vi "Port Number and Machine Name.vi"(0 "LV DEV in":refnum<class "LV DEV.lvclass">, 5 "PID":string, 11 "error in (no error)":errorcluster) -> (4 "LV DEV out":refnum<class "LV DEV.lvclass">, 6 "Machine Name":string, 8 "Port Number":u16, 15 "error out":errorcluster)   [LabVIEW 2016, in "LV DEV.lvclass"]
uses:
  LV DEV.lvclass
  <vilib>/regexp/Match Regular Expression.xnode
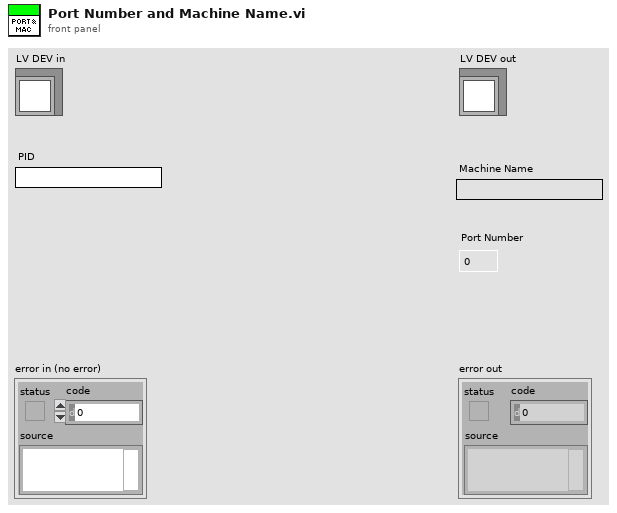
[diagram p1: front panel]
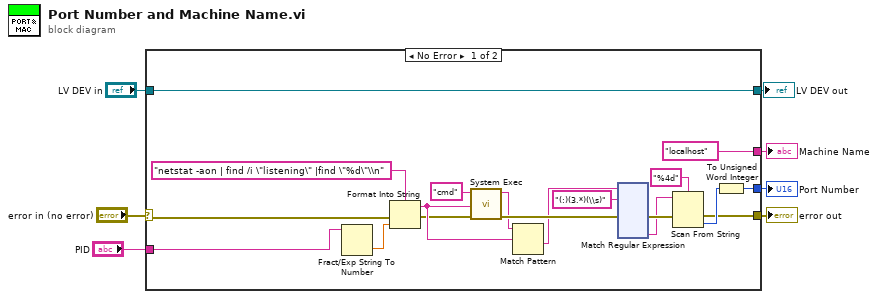
[diagram p0: block diagram]
diagram:
  n1 = case shown="No Error" "error in (no error)" {
    selector: "error in (no error)" -> [w12 w145]
    tunnel: [w11 w145] -> w6
    tunnel: "LV DEV in" -> [w26 w144]
    tunnel: [w26 w144] -> w4
    tunnel: "PID" -> [w10 _]
    tunnel: [w9 _] -> w2
    tunnel: ["localhost" _] -> w1
    frame No Error {
      n2 = Fract/Exp String To Number(string=w10) -> (number=w25:dbl)  [unwired: 3 in, 1 out]
      n3 = Format Into String(format string="netstat -aon | find /i \"listening\" |find \"%d\"\\n" ("standard input"), error in=w12, w25) -> (resulting string=w17:string, error out=w15:errorcluster)  [unwired: 1 in]
      n4 = call <vilib>:"System Exec.vi"("error in (no error)"=w15, "standard input"=w17, "command line"="cmd") -> ("error out"=w20:errorcluster, "standard output"=w16:string)  [unwired: 5 in, 2 out]
      n5 = Match Pattern(string=w16, regular expression=w17) -> (after substring=w18:string)  [unwired: 1 in, 3 out]
      n6 = xnode "Match Regular Expression"("input string"=w18, "regular expression"="(:)(3.*)(\\s)", "error in"=w20) -> ("error out"=w24:errorcluster, "submatch 2"=w21:string)  [unwired: 3 in, 5 out]
      n7 = Scan From String(format string="%4d", input string=w21, error in=w24) -> (error out=w11:errorcluster, output 1=w23:i32)  [unwired: 2 in, 2 out]
      n8 = To Unsigned Word Integer(number=w23) -> (unsigned 16bit integer=w9:u16)
    }
    frame Error {
    }
  }
  "error out" <- w6
  "LV DEV out" <- w4
  "Port Number" <- w2
  "Machine Name" <- w1
